vi "sg Query Pulse.vi"(8 "error in (no error)":errorcluster, 9 "width":dbl, 10 "period":dbl, 11 "device":i32) -> (0 "error out":errorcluster, 1 "width out":dbl, 2 "period out":dbl, 3 "function return":u32(ring))   [LabVIEW 2014, in "VSG25A.lvlib"]
doc: "SG_API sgStatus sgQueryPulse(int device, double *period, double *width);"
uses:
  VSG25A.lvlib
  sg_api.dll
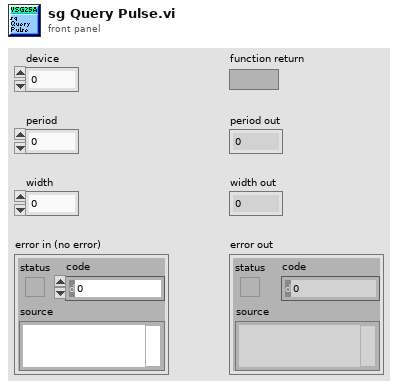
[diagram p1: front panel]
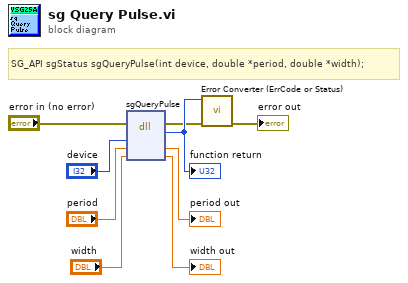
[diagram p0: block diagram]
diagram:
  # "SG_API sgStatus sgQueryPulse(int device, double *period, double *width);"
  n1 = dll-call lib="C:/Users/M_LAPTOP/Desktop/Labview/practice/VSG25A/sg_lib/sg_api.*" fn="sgQueryPulse"(error in="error in (no error)", "device"="device", "period"="period", "width"="width") -> (error out=w2:errorcluster, w9:u32, "period"=→"period out":dbl, "width"=→"width out":dbl)  [unwired: 3 in, 1 out]
  "function return" <- w9
  n2 = call "Error Converter (ErrCode or Status).vi"("error in (no error)"=w2, "error code"=w9) -> ("error out"=→"error out":errorcluster)  [unwired: 9 in]
